vi "ExportCallback.vi"(4 "User Parameter":T2, 6 "Control Ref":refnum<k24>, 7 "Event Common Data":T3) -> ()   [LabVIEW 2010]
uses:
  C:/BaseI/CodeBase/Applications/Assemblies/Spiricon.BeamGage.Automation.dll
  Applications/Assemblies/Spiricon.BeamGage.Automation.dll
  C:/BaseI/CodeBase/Applications/Assemblies/Spiricon.BeamGage.Automation.Interfaces.dll
  Applications/Assemblies/Spiricon.BeamGage.Automation.Interfaces.dll
panel:
  out "StartCapture":u32
  out "LoopNum":i32
  out "AExportStatusEnum":T1(ring)
  out "AExportStatus":i32
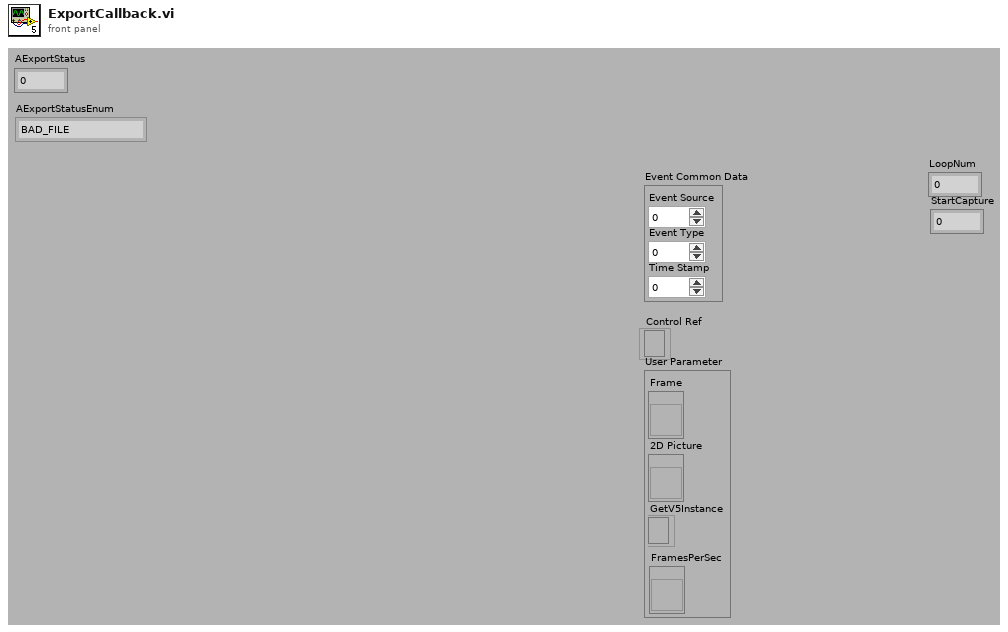
[diagram p1: front panel]
types:
  T1 = enum16{"BAD_FILE", "BAD_FRAME_NUM", "BASE_FILE_EXISTS", "BASE_FILE_IS_DIRECTORY", "GOOD", "NO_FILE_NAME", "NO_IMAGE", "READ_ONLY"}
  T2 = cluster{"Frame":refnum<vi>, "2D Picture":refnum<vi>, "GetV5Instance":refnum<k24>, "FramesPerSec":refnum<vi>}
  T3 = cluster{"Event Source":i32, "Event Type":u32, "Time Stamp":u32}
  T4 = typedef "imagedata.ctl" = cluster{"image type":i32, "image depth":i32, "image":u8[], "mask":u8[], "colors":u32[], "Rectangle":cluster{"left":i16, "top":i16, "right":i16, "bottom":i16}}
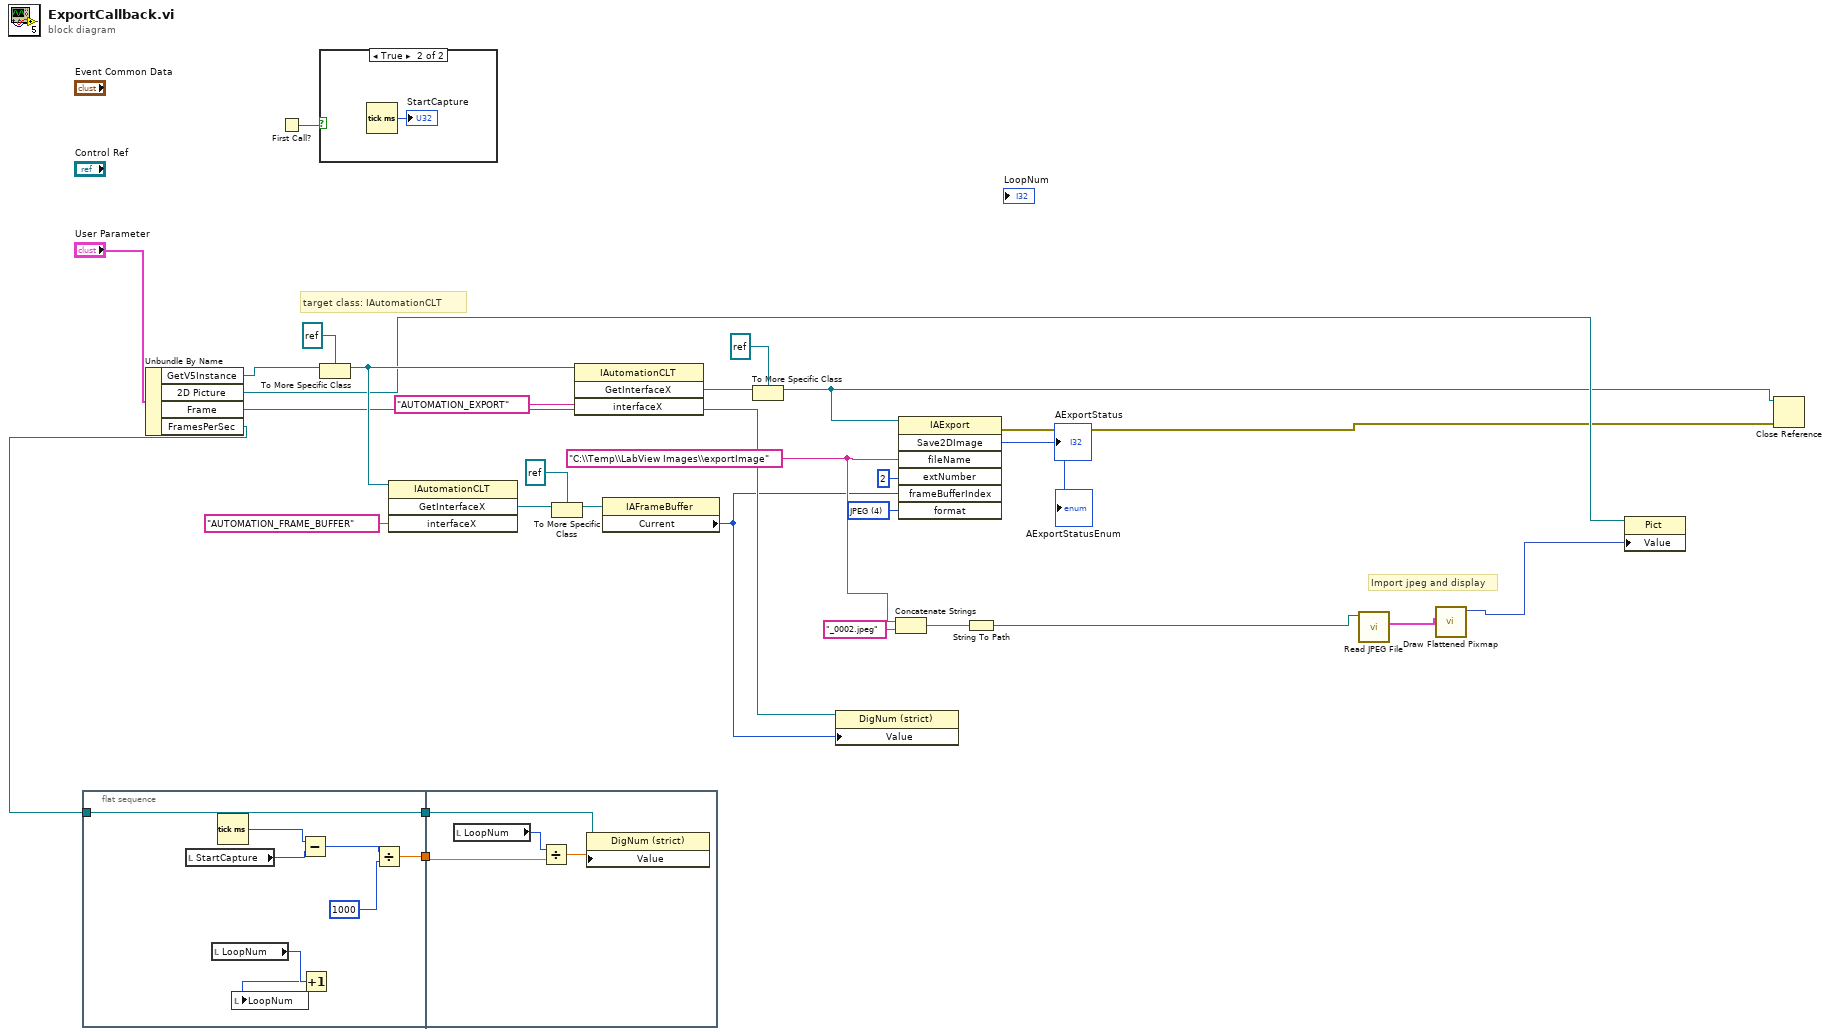
[diagram p0: block diagram]
diagram:
  w8 = 4 items=["NONE", "ASCII", "BMP", "GIF", "JPEG", "PNG", "TIFF"] ("format")
  w19 = "C:\\Temp\\LabView Images\\exportImage"
  # "Import jpeg and display"
  # "target class: IAutomationCLT"
  n1 = flat-sequence {
    tunnel: [w31] -> w13
    tunnel: w12 -> [w30]
    tunnel: [w30] -> w11
    tunnel: w13 -> [w40]
    tunnel: w11 -> [w39]
    frame #0 {
      n2 = local read "StartCapture"() -> (w32:u32)
      n3 = local read "LoopNum"() -> (w37:i32)
      n4 = Tick Count (ms)() -> (millisecond timer value=w33:u32)
      n5 = Subtract(x=w33, y=w32) -> (x-y=w34:u32)
      n6 = Increment(x=w37) -> (x+1=w36:i32)
      n7 = local write "LoopNum"(w36) -> ()
      n8 = Divide(x=w34, y=u32 1000 ("x-y")) -> (x/y=w31:dbl)
    }
    frame #1 {
      n9 = local read "LoopNum"() -> (w41:i32)
      n10 = Divide(x=w41, y=w40) -> (x/y=w38:dbl)
      n11 = property class="DigNum (strict)"(reference=w39, "Value"=w38) -> ()  [unwired: 1 in, 2 out]
    }
  }
  n12 = Unbundle By Name("User Parameter") -> ("GetV5Instance"=w20:refnum<k24>, "2D Picture"=w18:refnum<vi>, "Frame"=w17:refnum<vi>, "FramesPerSec"=w12:refnum<vi>)
  n13 = First Call?() -> (First Call?: T/F=w14:bool)
  n14 = case shown="True" w14 {
    frame False {
    }
    frame True {
      n15 = Tick Count (ms)() -> (millisecond timer value=→"StartCapture":u32)
    }
  }
  n16 = To More Specific Class(target class=refnum<k24> refnum, reference=w20) -> (specific class reference=w22:refnum<k24>)  [unwired: 1 in, 1 out]
  n17 = invoke class="IAutomationCLT" method="GetInterfaceX"(reference=w22, "interfaceX"="AUTOMATION_FRAME_BUFFER") -> ("GetInterfaceX"=w25:refnum<k24>)  [unwired: 2 in, 3 out]
  n18 = To More Specific Class(target class=refnum<k24> refnum, reference=w25) -> (specific class reference=w23:refnum<k24>)  [unwired: 1 in, 1 out]
  n19 = invoke class="IAutomationCLT" method="GetInterfaceX"(reference=w22, "interfaceX"="AUTOMATION_EXPORT") -> ("GetInterfaceX"=w27:refnum<k24>)  [unwired: 2 in, 3 out]
  n20 = property class="IAFrameBuffer"(reference=w23) -> ("Current"=w16:u32)  [unwired: 1 in, 2 out]
  n21 = To More Specific Class(target class=refnum<k24> refnum, reference=w27) -> (specific class reference=w10:refnum<k24>)  [unwired: 1 in, 1 out]
  n22 = property class="DigNum (strict)"(reference=w17, "Value"=w16) -> ()  [unwired: 1 in, 2 out]
  n23 = Concatenate Strings(w19, "_0002.jpeg" ("string")) -> (w4:string)
  n24 = invoke class="IAExport" method="Save2DImage"(reference=w10, "fileName"=w19, "extNumber"=u32 2, "frameBufferIndex"=w16, "format"=w8) -> (error out=w9:errorcluster, "Save2DImage"=→"AExportStatus" →"AExportStatusEnum":i32)  [unwired: 2 in, 5 out]
  n25 = String To Path(string=w4) -> (path=w3:path)
  n26 = call <vilib>:"Read JPEG File.vi"("path to JPEG file"=w3) -> ("image data"=w2:T4)  [unwired: 8 in, 2 out]
  n27 = call <vilib>:"Draw Flattened Pixmap.vi"("image data"=w2) -> ("new picture"=w1:picture)  [unwired: 8 in]
  n28 = property class="Pict"(reference=w18, "Value"=w1) -> ()  [unwired: 1 in, 2 out]
  n29 = Close Reference(reference=w10, error in (no error)=w9) -> ()  [unwired: 1 out]
